vi "Select DataBase.vi"(8 "error in (no error)":errorcluster, 11 "Database List":string[](array[string])) -> (0 "error out":errorcluster, 3 "Selected Database":string)   [LabVIEW 2017]
panel:
  in  "Select":bool
  in  "DataBase List":i32(listbox)
  # "SELECT DATA BASE"
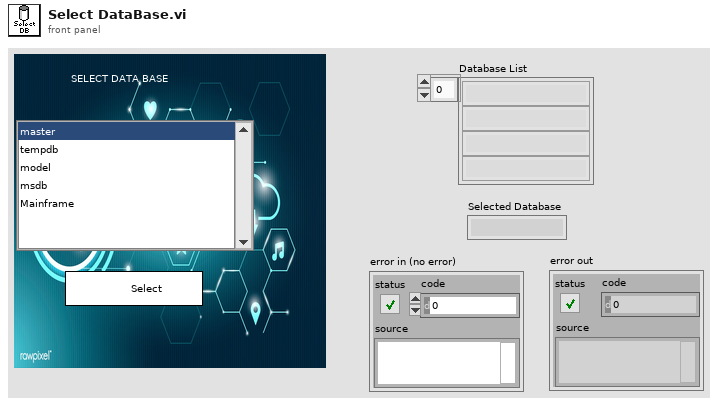
[diagram p1: front panel]
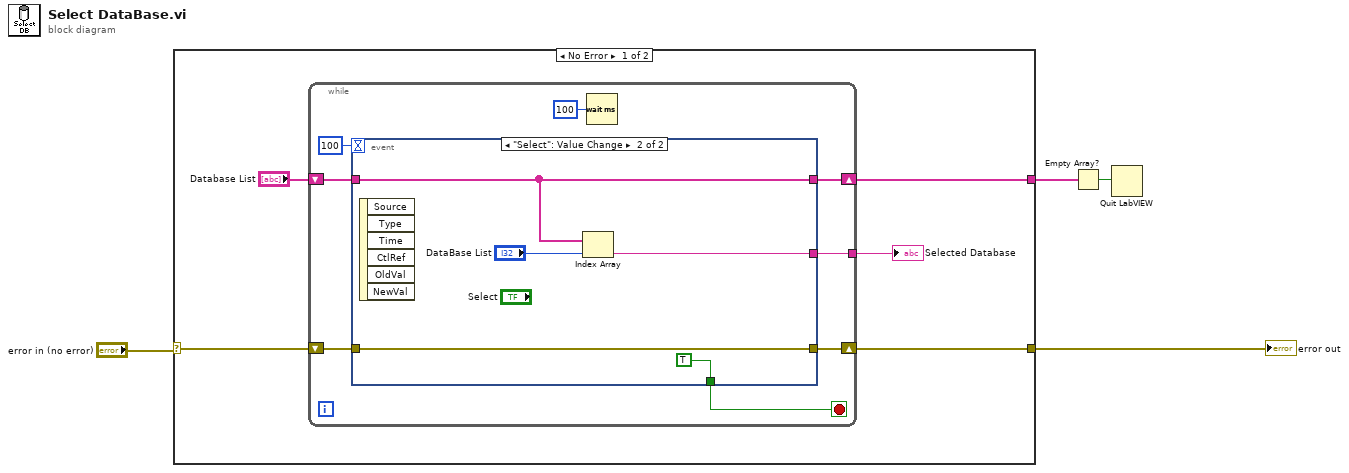
[diagram p0: block diagram]
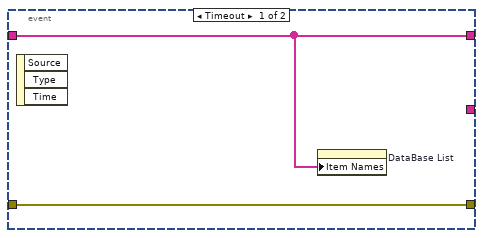
[diagram p2: hidden frame]
diagram:
  n1 = case shown="No Error" "error in (no error)" {
    selector: "error in (no error)" -> [w8 w25]
    tunnel: [w7 w25] -> w3
    tunnel: [w6 _] -> w2
    frame No Error {
      n2 = while {
        shift-right: [w16] -> w6
        shift-left: "Database List" -> [w15]
        tunnel: [w14] -> w9
        shift-right: [w10] -> w7
        shift-left: w8 -> [w11]
        stop <- w13 stop-if-true
        n3 = event shown="[1] \"Select\": Value Change" {
          selector: _ -> [_ _]
          dyn-events: _ -> [_ _]
          timeout: 100 -> [_ _]
          tunnel: [w18 w23] -> w16
          tunnel: w15 -> [w18 w23]
          tunnel: [_ w22] -> w14
          tunnel: [_ TRUE] -> w13
          tunnel: w11 -> [w19 w20]
          tunnel: [w19 w20] -> w10
          event Timeout {
            n4 = event-data() -> ()  [unwired: 1 in, 3 out]
            n5 = property on="DataBase List" class="LstBox (strict)"("Item Names"=w18) -> ()  [unwired: 2 in, 2 out]
          }
          event "Select": Value Change {
            n6 = event-data() -> ()  [unwired: 1 in, 6 out]
            n7 = Index Array(array=w23, index="DataBase List") -> (element=w22:string)
          }
        }
        n8 = Wait (ms)(milliseconds to wait=u32 100) -> ()  [unwired: 1 out]
      }
      "Selected Database" <- w9
    }
    frame Error {
    }
  }
  "error out" <- w3
  n9 = Empty Array?(array=w2) -> (empty?=w1:bool)
  n10 = Quit LabVIEW(quit? (T)=w1) -> ()
